vi "test Parse Sorted Object Dictionary_6.vi"(11 "Test Case In":refnum<class "test Electronic Datasheet.lvclass">) -> (0 "error out":errorcluster, 3 "Test Case Out":refnum<class "test Electronic Datasheet.lvclass">)   [LabVIEW 2024, in "test Electronic Datasheet.lvclass"]
uses:
  test Electronic Datasheet.lvclass
  C:/Program Files/National Instruments/LabVIEW 2024/vi.lib/Astemes/LUnit/Test Case.lvclass
  <vilib>/Astemes/LUnit/Test Case.lvclass/Test Case.ctl
  997a5cc8-28e7-4c8b-bc0c-c7deaea17f55.vi
  <vilib>/Astemes/LUnit/Append Pass Result.vi
  <vilib>/Astemes/LUnit/Append Fail Result.vi
  <vilib>/Astemes/LUnit/Describe Comparison.vi
  997a5cc8-28e7-4c8b-bc0c-c7deaea17f55.vi/9c5d11cd-9439-4240-a1ee-d9baace9c924.vi
  <vilib>/Astemes/LUnit/Run In UI.vi
  <vilib>/Utility/error.llb/Clear Errors.vi
  Electronic Datasheet/utils/Electronic Datasheet_GetAttributes.vi
  <vilib>/Astemes/LUnit/Describe Variant.vi
  test Electronic Datasheet.lvclass/test Electronic Datasheet.ctl
  Electronic Datasheet/Electronic Datasheet.lvclass
  Core/OD Entry/OD Entry.lvclass
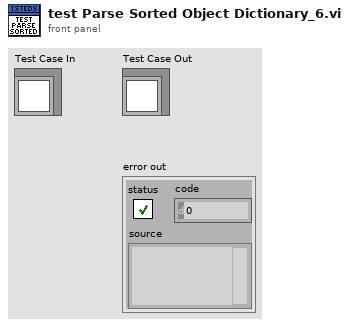
[diagram p1: front panel]
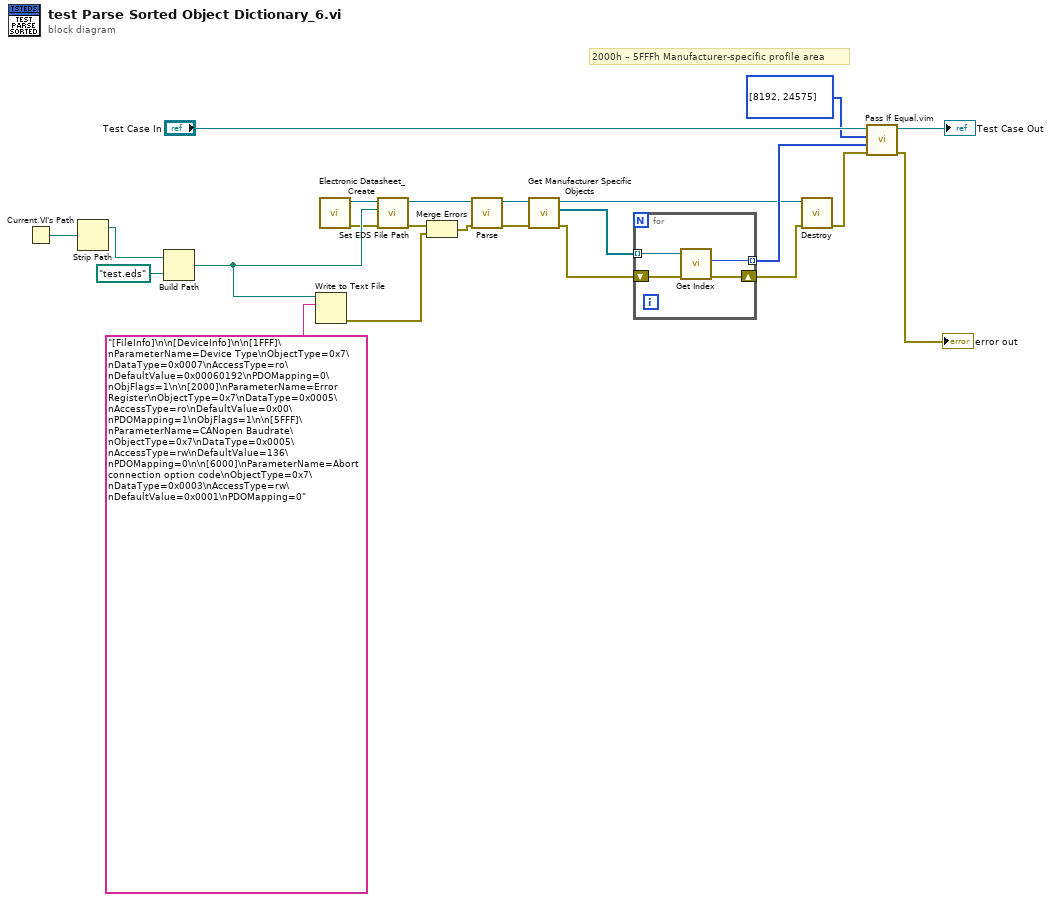
[diagram p0: block diagram]
diagram:
  # "2000h – 5FFFh Manufacturer-specific profile area"
  n1 = Current VI's Path() -> (path=w19:path)
  n2 = Strip Path(path=w19) -> (stripped path=w15:path)  [unwired: 1 out]
  n3 = Build Path(base path=w15, name or relative path=path "test.eds") -> (appended path=w16:path)
  n4 = Write to Text File(file (use dialog)=w16, text="[FileInfo]\n\n[DeviceInfo]\n\n[1FFF]\nParameterName=Device Type\nObjectType=0x7\nDataType=0x0007\nAccessType=ro\nDefaultValue=0x00060192\nPDOMapping=0\nObjFlags=1\n\n[2000]\nParameterName=Error Register\nObjectType=0x7\nDataType=0x0005\nAccessType=ro\nDefaultValue=0x00\nPDOMapping=1\nObjFlags=1\n\n[5FFF]\nParameterName=CANopen Baudrate\nObjectType=0x7\nDataType=0x0005\nAccessType=rw\nDefaultValue=136\nPDOMapping=0\n\n[6000]\nParameterName=Abort connection option code\nObjectType=0x7\nDataType=0x0003\nAccessType=rw\nDefaultValue=0x0001\nPDOMapping=0") -> (error out=w17:errorcluster)  [unwired: 2 in, 2 out]
  n5 = call "Electronic Datasheet_Create.vi"() -> ("Error Out"=w3:errorcluster, "reference out"=w4:refnum<class "Electronic Datasheet.lvclass">)  [unwired: 10 in]
  n6 = call "Set EDS File Path.vi"("error in"=w3, "EDS File Path"=w16, "reference in"=w4) -> ("error out"=w1:errorcluster, "reference out"=w20:refnum<class "Electronic Datasheet.lvclass">)  [unwired: 7 in]
  n7 = Merge Errors(w1, w17) -> (w2:errorcluster)
  n8 = call "Parse.vi"("error in"=w2, "reference in"=w20) -> ("error out"=w12:errorcluster, "reference out"=w8:refnum<class "Electronic Datasheet.lvclass">)  [unwired: 8 in]
  n9 = call "Get Manufacturer Specific Objects.vi"("error in"=w12, "reference in"=w8) -> ("error out"=w6:errorcluster, "Entries"=w11:refnum<class "OD Entry.lvclass">[], "reference out"=w7:refnum<class "Electronic Datasheet.lvclass">)  [unwired: 7 in]
  n10 = for {
    tunnel: w11 -> [w27] mode=indexing
    tunnel: [w26] -> w9 mode=indexing
    shift-right: [w24] -> w5
    shift-left: w6 -> [w25]
    n11 = call "Get Index.vi"("Error In"=w25, "reference in"=w27) -> ("Error Out"=w24:errorcluster, "Index"=w26:u16)  [unwired: 7 in, 1 out]
  }
  n12 = call-dynamic "Destroy.vi"("Error In"=w5, "reference in"=w7) -> ("Error Out"=w13:errorcluster)  [unwired: 8 in, 1 out]
  n13 = call "Pass If Equal.vim"("error in (no error)"=w13, "Actual"=w9, "Expected"=u16[] [8192, 24575] ("Array"), "LUnit Test Case In"="Test Case In") -> ("error out"=→"error out":errorcluster, "LUnit Test Case Out"=→"Test Case Out":refnum<class "test Electronic Datasheet.lvclass">)  [unwired: 6 in]
